vi "OrientationToTarget.vi"(9 "Robot Y":dbl, 10 "Robot X":dbl, 11 "Robot Orientation":dbl) -> ()   [LabVIEW 2018]
panel:
  out "Target":string
  in  "Target In Sight":bool
  # "CR"
  # "CL"
  # "Naming Convention: [R, C, P], [L, R],[T, M, B, L, R] \n[Rocket, Cargo Ship, or Player Station] + [Left, or Right of field] + [Top, Middle, Bottom, Left, Right, or Down]"
  # "X, 0"
  # "x,y"
  # "CLT"
  # "CRT"
  # "CLM"
  # "CRM"
  # "Note, the value of the third piece of the name for the player station should be Bottom, regardless of anything else\nand also, the bottom facing cargo targets have the \"Down\" designation"
  # "RRT"
  # "RLT"
  # "CLB"
  # "CRB"
  # "See the picture to the left for the names of each target (they are in black so a bit hard to see, sorry)\nAlso, please see the INSTRUCTIONS below:"
  # "RRM"
  # "INSTRUCTIONS: Thank you a bunch for helping me code this stuff. I know this task is a bit tedious, but it is extremely important. This is file is part of how we will decide what target we are looking at to plan a path to drive towards!! Please read this entire piece of text before you begin.\n\n1) Your goal today is to make this VI perform its job. What job?? Well, you are gonna take the three provided inputs, Approximate X, Approximate Y,  Orientation, and a boolean telling you whether there is a target in sight or not,  and return the orientation of the target the camera is seeing, relative to the field. HOW????? Well, hopefully these instructions will help.\n\n2) First off, note the coordinate frame that exists in the four corners of the attatched image! That is your x,y frame. Also note that the orientation is 0 along the x axis and 90 along the y axis. However, the input robot orientation is 0 facing upwards, along the y-axis. Please keep this in mind when you are designing.\n\n3) Start by creating a google sheet (which you should share with me), that lists the name, x, y, orientation (relative to the field so if it is horizontal and facing left, then it is at 0 degrees), and height of each target. If the target has more than one height (like the cargo ship), then put the height of the hatch. These values should be between 2,7 feet and 3,6 feet but that is NOT exact: you need to reference the game manual. This google sheet will be used later for other things, and will be the MOST important part of my ENTIRE project. If the values in that are not accurate, nothing related to vision will work. Please be dilligent when filling out the document. I know it is boring. If you want help, come find someone to help you. I really appreciate it.\n\n4) Once you have the sheet, the fun stuff begins!! Well . . . kinda fun. ish. Ok, so first, determine what quadrant of the field the robot is \"in\". Then for each quadrant case, add four cases for four general orientations, \"up\", \"left\", \"right\", \"down\". Remember, the robot orientation starts with 0 facing upwards. make the ranges 90 degrees each. Now, you should have 16 cases.  For each case, use the passed in boolean to make another case: target in sight, or target not in sight. Note here that the horizontal fov of the camera is 52 degrees: that number may or may not influence how you break up the various quadrants and orientations. Go through each case, and think about what orientation a target in sight would be. Remember, even if there are multiple targets in sight, chances are that they will all be facing the same direction. We only need the orientation of the target, and there are only 6 possibilities (left, right, up, down, angled up, angled down). For each case, output the most likely orientation of the target. For cases where no targets are in sight, but should be, put a comment. Do the same for cases where there are targets in sight but shouldn't be. That should cover every case, and you would be done with this project.\n\n5) If you have any questions and can't figure the answers out, come to me. This is not a trivial task, and is quite tedious: my apologies for that, especially since I am pretty much throwing you into the deep end. I really appreciate it, this will go a long way towards helping the team win!! Also, don't worry about finishing everything today, but try and get any questions out today, since I will not be there Thursday."
  # "RLM"
  # "CB"
  # "CLD"
  # "CRD"
  # "RLB"
  # "RRB"
  # "PLB"
  # "PRB"
  # "0,Y"
  # "0, 0"
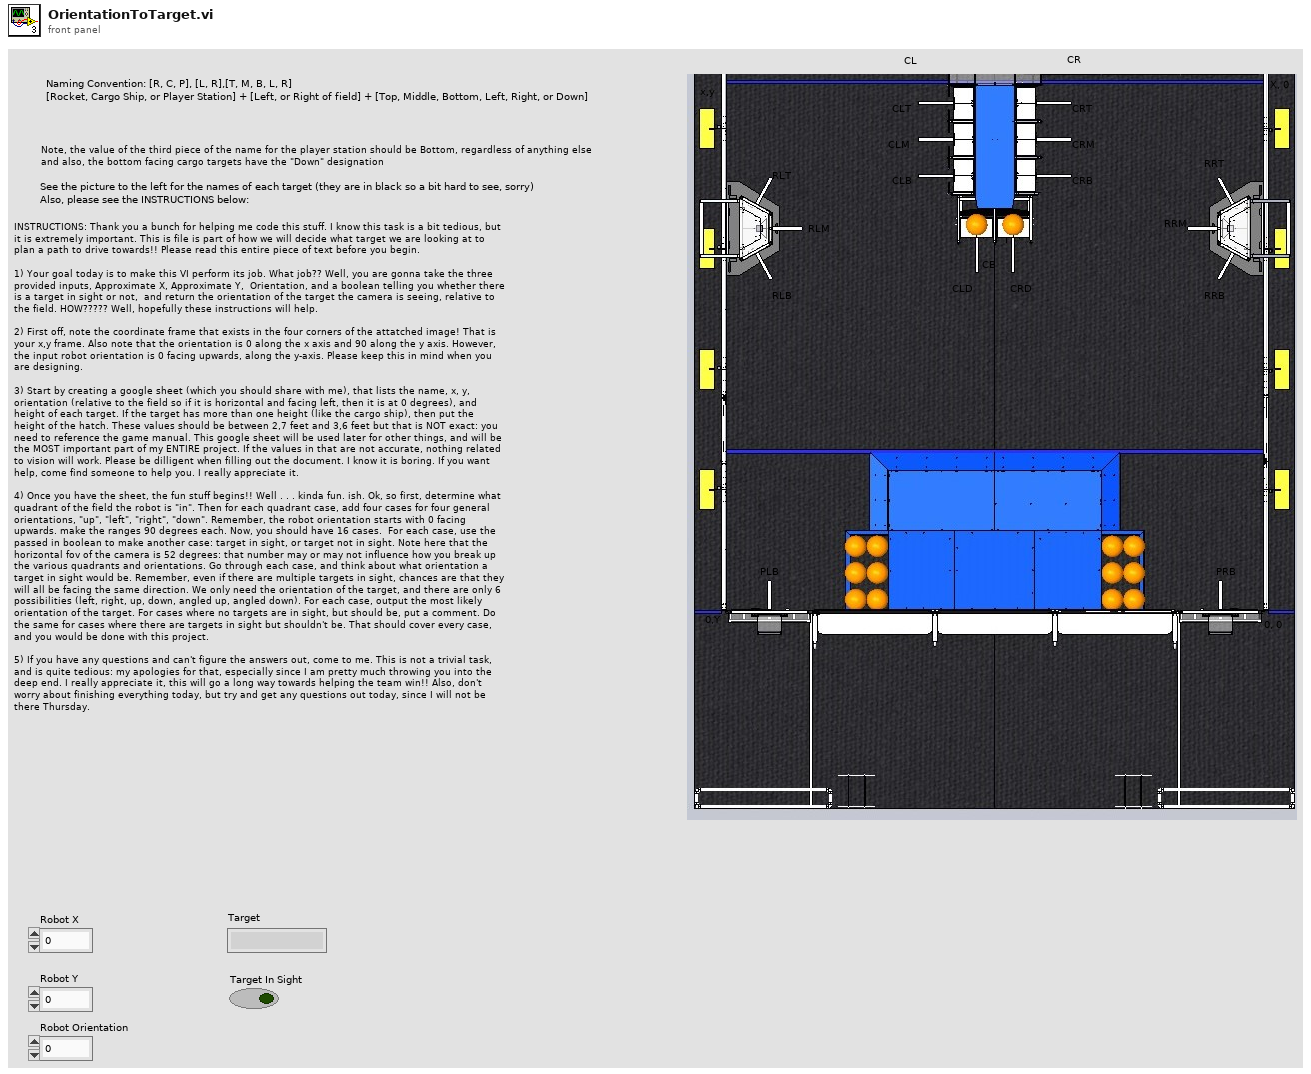
[diagram p1: front panel]
types:
  T1 = typedef "TargetDataType.ctl" = cluster{"Name":string, "x":dbl, "y":dbl, "orientation":dbl, "height":dbl}
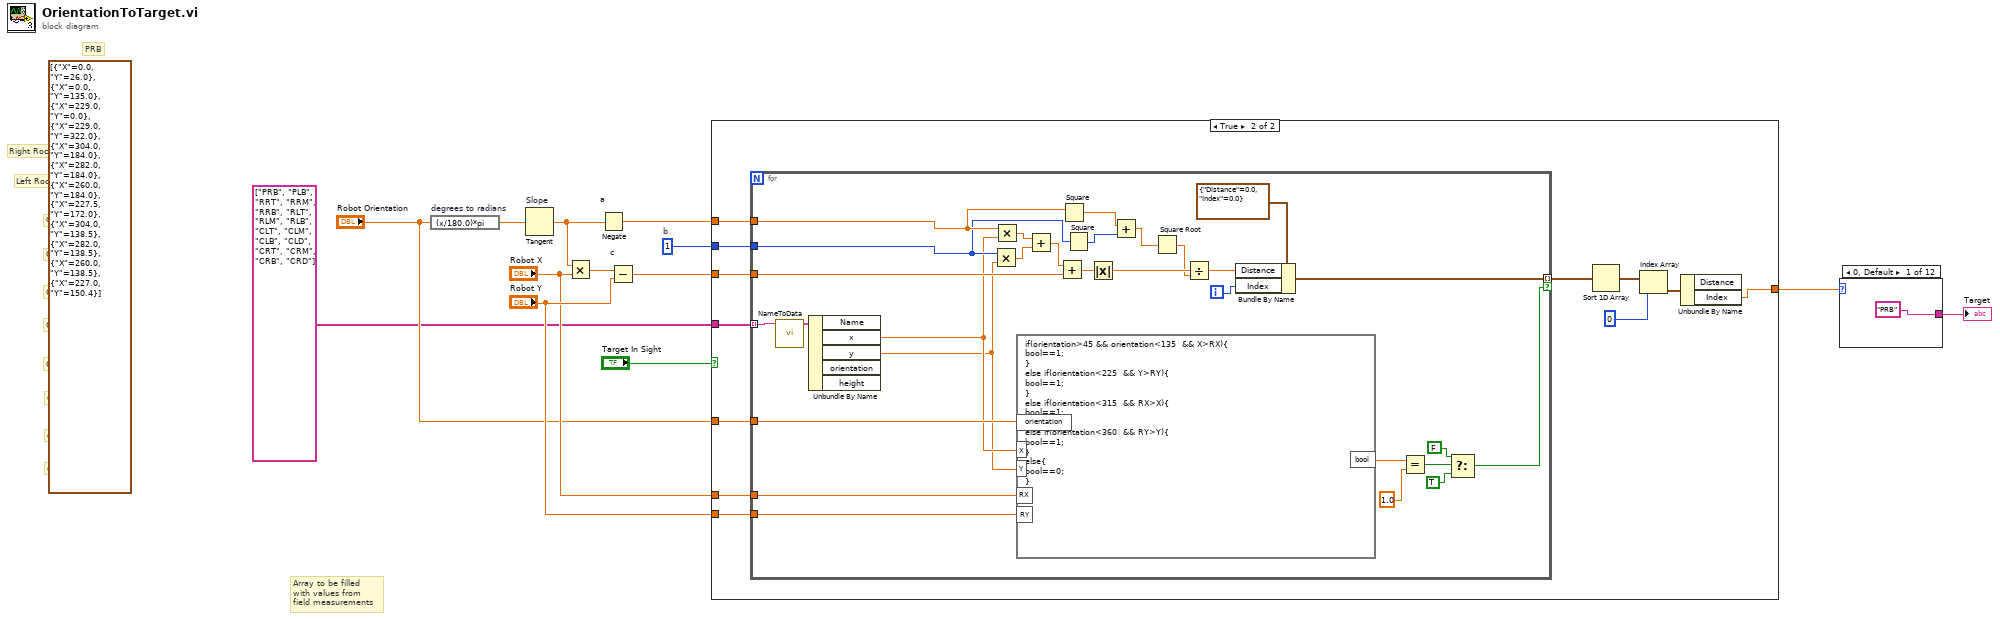
[diagram p0: block diagram]
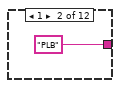
[diagram p2: hidden frame]
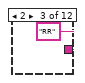
[diagram p3: hidden frame]
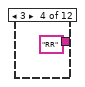
[diagram p4: hidden frame]
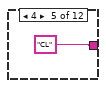
[diagram p5: hidden frame]
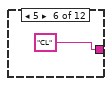
[diagram p6: hidden frame]
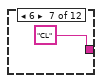
[diagram p7: hidden frame]
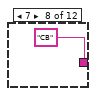
[diagram p8: hidden frame]
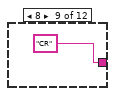
[diagram p9: hidden frame]
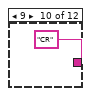
[diagram p10: hidden frame]
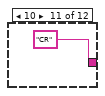
[diagram p11: hidden frame]
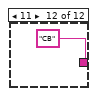
[diagram p12: hidden frame]
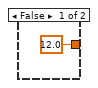
[diagram p13: hidden frame]
diagram:
  (unwired) cluster{"X":dbl, "Y":dbl}[] [{"X"=0.0, "Y"=26.0}, {"X"=0.0, "Y"=135.0}, {"X"=229.0, "Y"=0.0}, {"X"=229.0, "Y"=322.0}, {"X"=304.0, "Y"=184.0}, {"X"=282.0, "Y"=184.0}, {"X"=260.0, "Y"=184.0}, {"X"=227.5, "Y"=172.0}, {"X"=304.0, "Y"=138.5}, {"X"=282.0, "Y"=138.5}, {"X"=260.0, "Y"=138.5}, {"X"=227.0, "Y"=150.4}]
  w9 = 1  # b
  # "CRD"
  # "CRB"
  # "CRM"
  # "CRT"
  # "CLD"
  # "CLB"
  # "CLM"
  # "CLT"
  # "Left Rocket"
  # "Right Rocket"
  # "PLB"
  # "Array to be filled\nwith values from \nfield measurements"
  # "PRB"
  n1 = expression code="(x/180.0)*pi" "degrees to radians"("Robot Orientation") -> (w3:dbl)
  n2 = Tangent "Slope"(1:w3) -> (0:w12:dbl)
  n3 = Multiply(x=w12, y="Robot X") -> (x*y=w11:dbl)
  n4 = Negate "a"(x=w12) -> (-x=w10:dbl)
  n5 = Subtract "c"(x=w11, y="Robot Y") -> (x-y=w8:dbl)
  n6 = case shown="True" "Target In Sight" {
    tunnel: w10 -> [_ w25]
    tunnel: w9 -> [_ w24]
    tunnel: w8 -> [_ w23]
    tunnel: string[] ["PRB", "PLB", "RRT", "RRM", "RRB", "RLT", "RLM", "RLB", "CLT", "CLM", "CLB", "CLD", "CRT", "CRM", "CRB", "CRD"] -> [_ w26]
    tunnel: "Robot Orientation" -> [_ w22]
    tunnel: "Robot Y" -> [_ w21]
    tunnel: "Robot X" -> [_ w20]
    tunnel: [12.0 ("Index") w15] -> w5
    frame False {
    }
    frame True {
      n7 = for {
        tunnel: w26 -> [w30] mode=indexing
        tunnel: w25 -> [w49]
        tunnel: w24 -> [w48]
        tunnel: w23 -> [w52]
        tunnel: [w40] -> w19 mode=indexing if=w31
        tunnel: w22 -> [w39]
        tunnel: w21 -> [w38]
        tunnel: w20 -> [w37]
        i -> [w42]
        n8 = call "NameToData.vi"("Name"=w30) -> ("Target"=w29:T1)  [unwired: 10 in]
        n9 = Unbundle By Name(w29) -> ("x"=w28:dbl, "y"=w27:dbl)  [unwired: 3 out]
        n10 = Multiply(x=w48, y=w27) -> (x*y=w54:dbl)
        n11 = Multiply(x=w49, y=w28) -> (x*y=w55:dbl)
        n12 = formula code="if(orientation>45 && orientation<135  && X>RX){\nbool==1;\n}\nelse if(orientation<225  && Y>RY){\nbool==1;\n}\nelse if(orientation<315  && RX>X){\nbool==1;\n}\nelse if(orientation<360  && RY>Y){\nbool==1;\n}\nelse{\nbool==0;\n}"("orientation"=w39, "X"=w28, "Y"=w27, "RX"=w37, "RY"=w38) -> ("bool"=w36:dbl)
        n13 = Add(x=w55, y=w54) -> (x+y=w53:dbl)
        n14 = Add(x=w53, y=w52) -> (x+y=w51:dbl)
        n15 = Square(x=w49) -> (x^2=w46:dbl)
        n16 = Square(x=w48) -> (x^2=w47:i32)
        n17 = Absolute Value(x=w51) -> (abs(x)=w50:dbl)
        n18 = Add(x=w46, y=w47) -> (x+y=w45:dbl)
        n19 = Square Root(x=w45) -> (sqrt(x)=w44:dbl)
        n20 = Divide(x=w50, y=w44) -> (x/y=w41:dbl)
        n21 = Bundle By Name(cluster=cluster{"Distance":dbl, "Index":dbl} {"Distance"=0.0, "Index"=0.0}, "Distance"=w41, "Index"=w42) -> (w40:cluster{"Distance":dbl, "Index":dbl})
        n22 = Equal?(x=w36, y=1.0) -> (x = y?=w34:bool)
        n23 = Select(t=FALSE, s=w34, f=TRUE) -> (s? t:f=w31:bool)
      }
      n24 = Sort 1D Array(array=w19) -> (sorted array=w18:cluster{"Distance":dbl, "Index":dbl}[])
      n25 = Index Array(array=w18, index=0) -> (element=w16:cluster{"Distance":dbl, "Index":dbl})
      n26 = Unbundle By Name(w16) -> ("Index"=w15:dbl)  [unwired: 1 out]
    }
  }
  n27 = case shown="0, Default" w5 {
    tunnel: ["PRB" ("Target") "PLB" ("Target") "RR" ("Target") "RR" ("Target") "CL" ("Target") "CL" ("Target") "CL" ("Target") "CB" ("Target") "CR" ("Target") "CR" ("Target") "CR" ("Target") "CB" ("Target")] -> w4
    frame 0, Default {
    }
    frame 1 {
    }
    frame 2 {
    }
    frame 3 {
    }
    frame 4 {
    }
    frame 5 {
    }
    frame 6 {
    }
    frame 7 {
    }
    frame 8 {
    }
    frame 9 {
    }
    frame 10 {
    }
    frame 11 {
    }
  }
  "Target" <- w4
